vi "queuefr.vi"() -> ()   [LabVIEW 2015]
uses:
  enum.ctl
panel:
  out "Numeric 2":i32
  out "ButtonInCluster":string[](array[string])
  in  "離開":bool
  in  "Action10":bool
  in  "Action9":bool
  in  "Action8":bool
  in  "Action7":bool
  in  "Action6":bool
  in  "Action5":bool
  in  "Action4":bool
  in  "Action3":bool
  in  "Action2":bool
  out "ButtonOnVI":string[](array[string])
  in  "Action1":bool
  in  "初始化":bool
  in  "Enum":T1
  out "element":T1
  in  "Cluster":T2
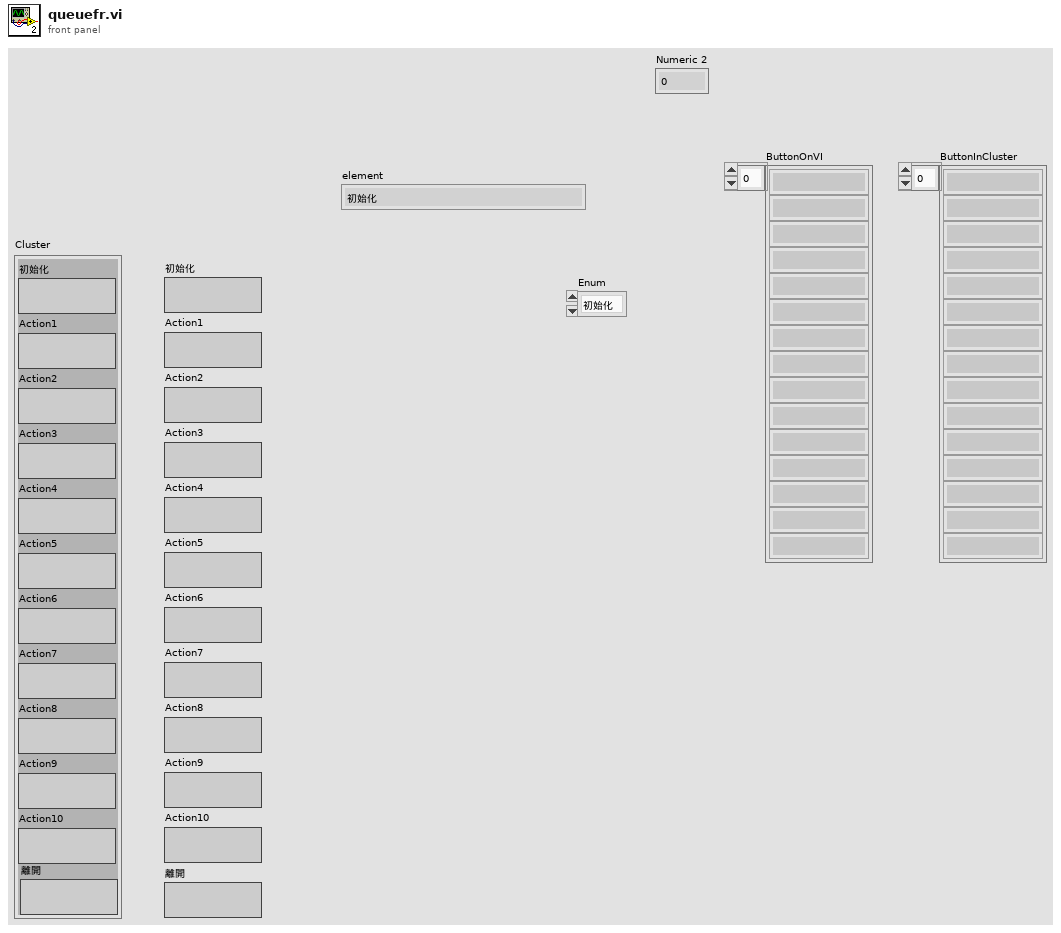
[diagram p1: front panel]
types:
  T1 = typedef "enum.ctl" = enum16{"初始化", "等待", "離開", "Action1", "Action2", "Action3", "Action4", "Action5", "Action6", "Action7", "Action8", "Action9", "Action10"}
  T2 = cluster{"初始化":bool, "Action1":bool, "Action2":bool, "Action3":bool, "Action4":bool, "Action5":bool, "Action6":bool, "Action7":bool, "Action8":bool, "Action9":bool, "Action10":bool, "離開":bool}
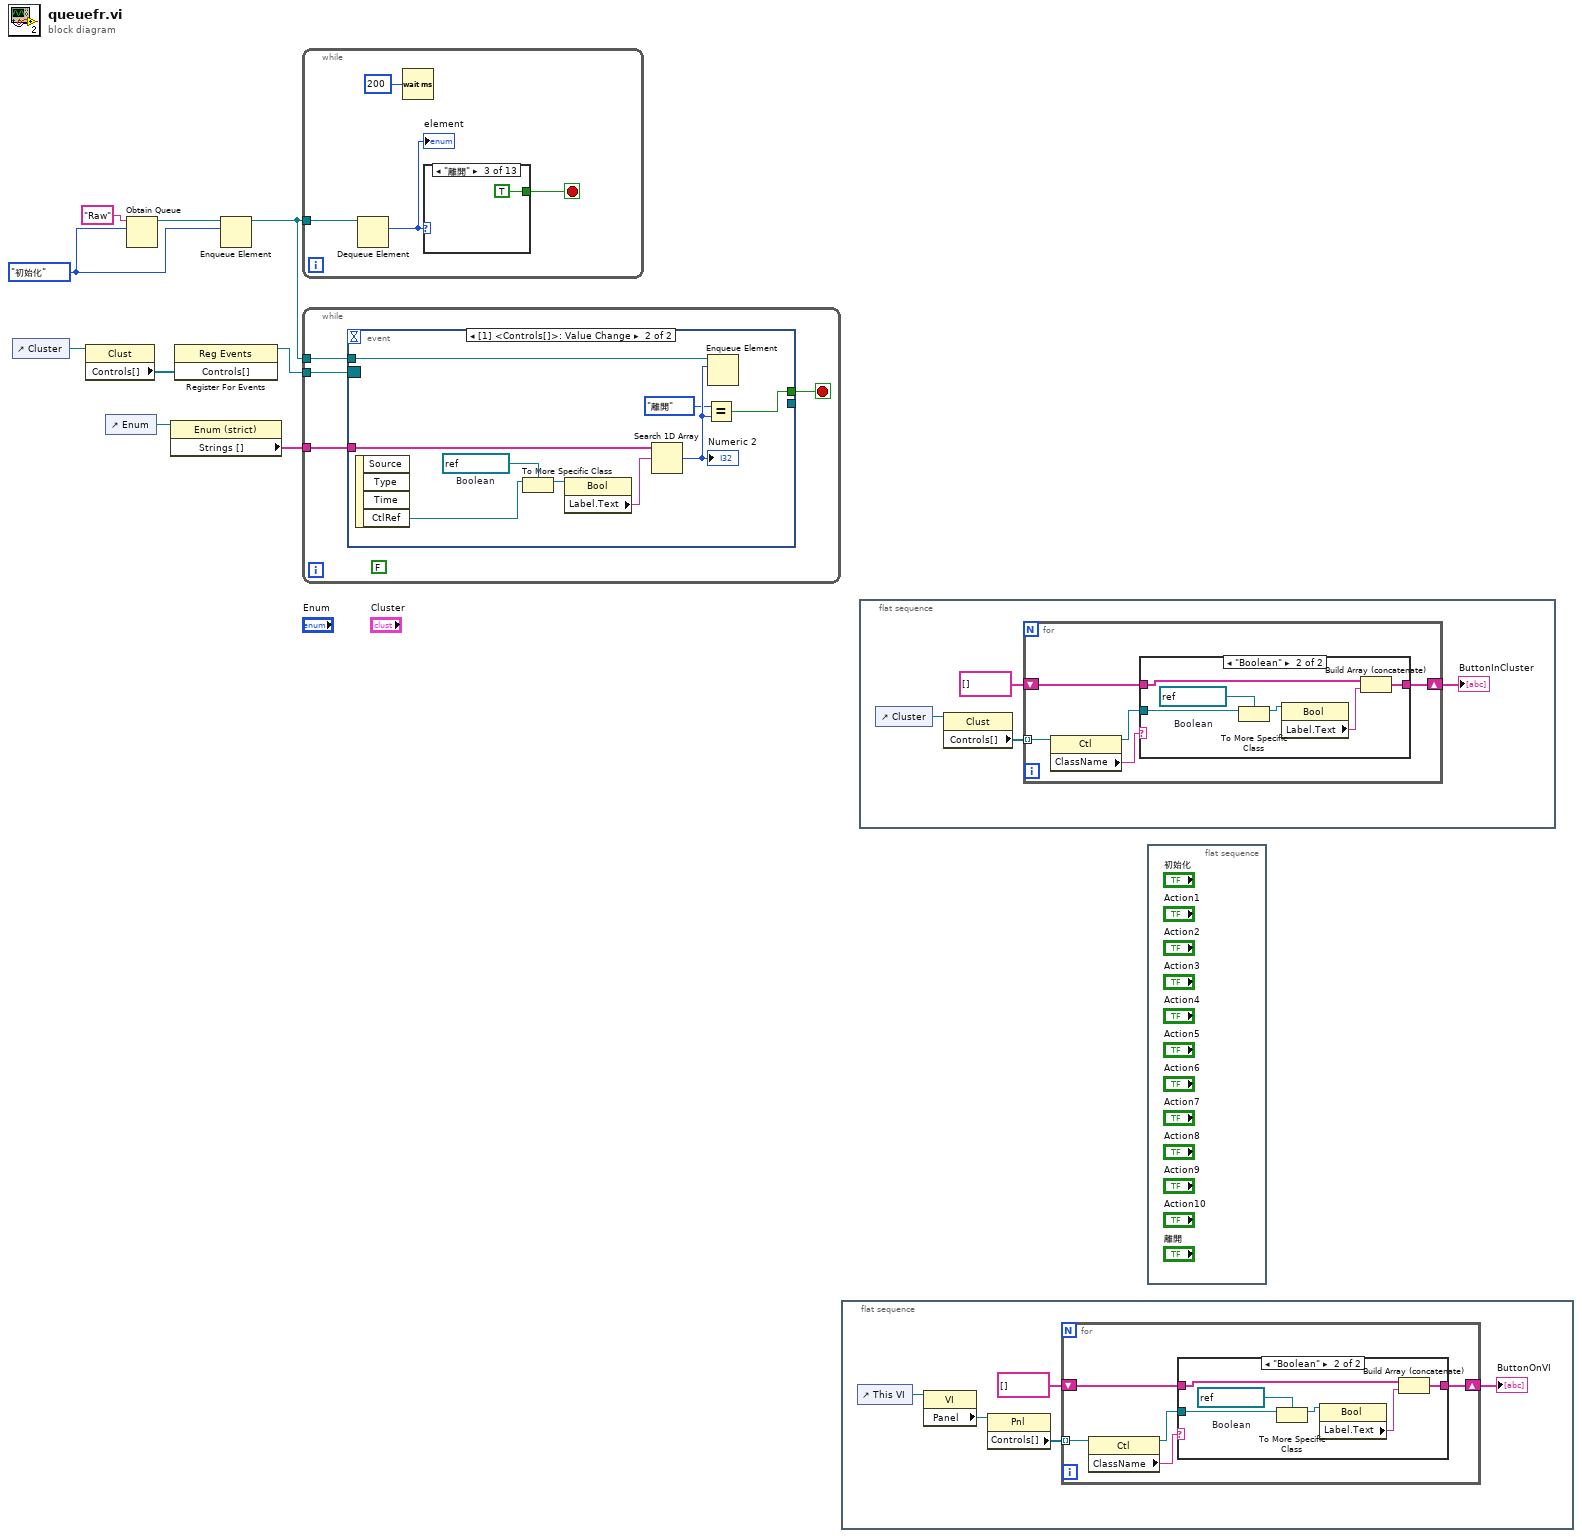
[diagram p0: block diagram]
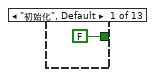
[diagram p4: hidden frame]
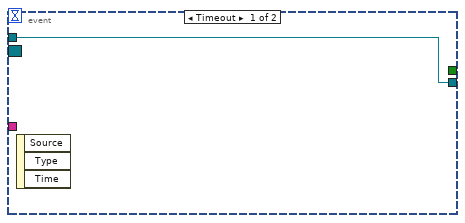
[diagram p16: hidden frame]
diagram:
  w7 = enum."初始化" ("Enum")
  n1 = control-ref of="Cluster"() -> (w2:refnum<vi>)
  n2 = property class="Clust"(reference=w2) -> ("Controls[]"=w1:refnum<vi>[])  [unwired: 1 in, 2 out]
  n3 = control-ref of="Enum"() -> (w4:refnum<vi>)
  n4 = Obtain Queue(name (unnamed)="Raw", element data type=w7) -> (queue out=w9:refnum<queue>)  [unwired: 3 in, 2 out]
  n5 = property class="Enum (strict)"(reference=w4) -> ("Strings []"=w3:string[])  [unwired: 1 in, 2 out]
  n6 = register-events(w1) -> (reference out=w5:refnum<event-registration>)  [unwired: 2 in, 1 out]
  n7 = Enqueue Element(queue=w9, element=w7) -> (queue out=w6:refnum<queue>)  [unwired: 2 in, 2 out]
  n8 = while {
    tunnel: w6 -> [w13]
    stop <- w11 stop-if-true
    n9 = Dequeue Element(queue=w13) -> (element=w12:T1)  [unwired: 2 in, 3 out]
    "element" <- w12
    n10 = Wait (ms)(milliseconds to wait=u32 200) -> ()  [unwired: 1 out]
    n11 = case shown="\"離開\"" w12 {
      tunnel: [FALSE _ TRUE _ _ _ _ _ _ _ _ _ _] -> w11
      frame "初始化", Default {
      }
      frame "等待" {
      }
      frame "離開" {
      }
      frame "Action1" {
      }
      frame "Action2" {
      }
      frame "Action3" {
      }
      frame "Action4" {
      }
      frame "Action5" {
      }
      frame "Action6" {
      }
      frame "Action7" {
      }
      frame "Action8" {
      }
      frame "Action9" {
      }
      frame "Action10" {
      }
    }
  }
  n12 = while {
    tunnel: w6 -> [w19]
    tunnel: w5 -> [w18]
    tunnel: w3 -> [w17]
    stop <- w16 stop-if-true
    (unwired) FALSE
    n13 = event shown="[1] <Controls[]>: Value Change" {
      selector: w18 -> [_ _]
      dyn-events: _ -> [_ _]
      timeout: _ -> [_ _]
      tunnel: [w20 _] -> _
      tunnel: w19 -> [w20 w26]
      tunnel: w17 -> [_ w25]
      tunnel: [_ w21] -> w16
      event Timeout {
        n14 = event-data() -> ()  [unwired: 1 in, 3 out]
      }
      event Value Change {
        w29 = refnum<vi> refnum  # Boolean
        n15 = event-data() -> ("CtlRef"=w27:refnum<vi>)  [unwired: 1 in, 3 out]
        n16 = To More Specific Class(target class=w29, reference=w27) -> (specific class reference=w28:refnum<vi>)  [unwired: 1 in, 1 out]
        n17 = property class="Bool"(reference=w28) -> ("Label.Text"=w24:string)  [unwired: 1 in, 2 out]
        n18 = Search 1D Array(1D array=w25, element=w24) -> (index of element=w23:i32)  [unwired: 1 in]
        "Numeric 2" <- w23
        n19 = Equal?(x=enum."離開" ("Enum"), y=w23) -> (x = y?=w21:bool)
        n20 = Enqueue Element(queue=w26, element=w23) -> ()  [unwired: 2 in, 3 out]
      }
    }
  }
  n21 = flat-sequence {
    frame #0 {
      n22 = control-ref of="This VI"() -> (w32:refnum<vi>)
      n23 = property class="VI"(reference=w32) -> ("Panel"=w34:refnum<vi>)  [unwired: 1 in, 2 out]
      n24 = property class="Pnl"(reference=w34) -> ("Controls[]"=w33:refnum<vi>[])  [unwired: 1 in, 2 out]
      n25 = for {
        tunnel: w33 -> [w39] mode=indexing
        shift-right: [w36] -> w31
        shift-left: string[] [] -> [w35]
        n26 = property class="Ctl"(reference=w39) -> (reference out=w37:refnum<vi>, "ClassName"=w38:string)  [unwired: 1 in, 1 out]
        n27 = case shown="\"Boolean\"" w38 {
          tunnel: w37 -> [_ w44]
          tunnel: [w40 w43] -> w36
          tunnel: w35 -> [w40 w41]
          frame "False", Default {
          }
          frame "Boolean" {
            w46 = refnum<vi> refnum  # Boolean
            n28 = To More Specific Class(target class=w46, reference=w44) -> (specific class reference=w45:refnum<vi>)  [unwired: 1 in, 1 out]
            n29 = property class="Bool"(reference=w45) -> ("Label.Text"=w42:string)  [unwired: 1 in, 2 out]
            n30 = Build Array (concatenate)(w41, w42) -> (w43:string[])
          }
        }
      }
      "ButtonOnVI" <- w31
    }
  }
  n31 = flat-sequence {
    frame #0 {
      n32 = control-ref of="Cluster"() -> (w50:refnum<vi>)
      n33 = property class="Clust"(reference=w50) -> ("Controls[]"=w49:refnum<vi>[])  [unwired: 1 in, 2 out]
      n34 = for {
        tunnel: w49 -> [w55] mode=indexing
        shift-right: [w52] -> w47
        shift-left: string[] [] -> [w51]
        n35 = property class="Ctl"(reference=w55) -> (reference out=w53:refnum<vi>, "ClassName"=w54:string)  [unwired: 1 in, 1 out]
        n36 = case shown="\"Boolean\"" w54 {
          tunnel: w53 -> [_ w60]
          tunnel: [w56 w59] -> w52
          tunnel: w51 -> [w56 w57]
          frame "False", Default {
          }
          frame "Boolean" {
            w62 = refnum<vi> refnum  # Boolean
            n37 = To More Specific Class(target class=w62, reference=w60) -> (specific class reference=w61:refnum<vi>)  [unwired: 1 in, 1 out]
            n38 = property class="Bool"(reference=w61) -> ("Label.Text"=w58:string)  [unwired: 1 in, 2 out]
            n39 = Build Array (concatenate)(w57, w58) -> (w59:string[])
          }
        }
      }
      "ButtonInCluster" <- w47
    }
  }
  n40 = flat-sequence {
    frame #0 {
    }
  }
